vi "Deadband SubVI.vi"(1 "Joystick Value In":dbl) -> (0 "Joystick Value Out":dbl)   [LabVIEW 2014]
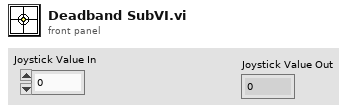
[diagram p1: front panel]
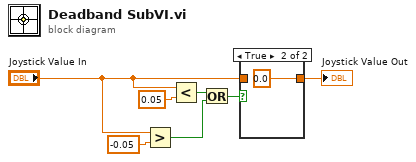
[diagram p0: block diagram]
diagram:
  n1 = Greater?(x="Joystick Value In", y=-0.05) -> (0:w4:bool)
  n2 = Less?(x="Joystick Value In", y=0.05 ("x")) -> (x < y?=w5:bool)
  n3 = Or(x=w5, y=w4) -> (x .or. y?=w3:bool)
  n4 = case shown="True" w3 {
    tunnel: [w8 0.0 ("y")] -> w1
    tunnel: "Joystick Value In" -> [w8 _]
    frame False {
    }
    frame True {
    }
  }
  "Joystick Value Out" <- w1
